vi "Set Cursor Busy.vi"(8 "error in (no error)":errorcluster, 10 "Disable Click?":bool, 11 "IViewable In":refnum<class "IViewable.lvclass">) -> (0 "error out":errorcluster, 3 "IViewable Out":refnum<class "IViewable.lvclass">)   [LabVIEW 2015, in "IViewable.lvlib" / "IViewable.lvclass"]
doc: "<License>\nCopyright © 2017 Composed Systems, LLC | All rights reserved\nwww.composed.io\n\nAuthor: Ethan Stern <ethan.stern@composed.io>\n\nThis software is provided \"AS IS\" WITHOUT WARRANTIES, either express or implied, AND IS FOR EDUCATIONAL PURPOSES ONLY.\n</License>"
uses:
  IViewable.lvclass
  IViewable.lvclass/IViewable.ctl
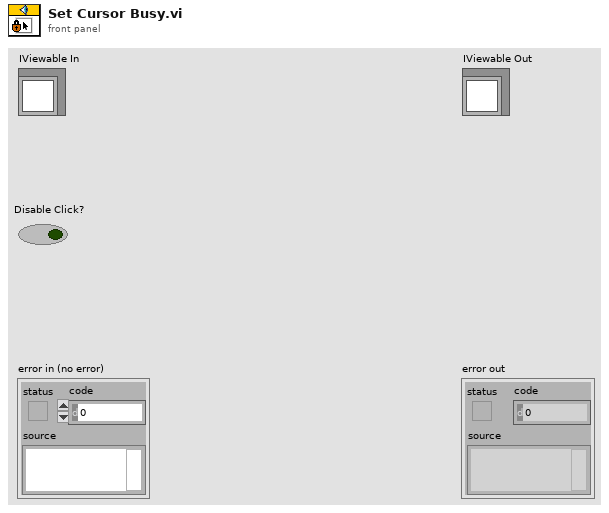
[diagram p1: front panel]
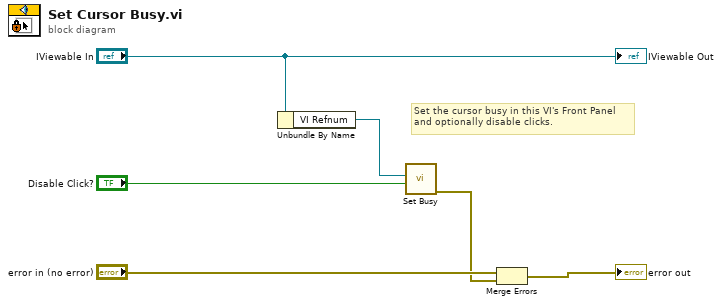
[diagram p0: block diagram]
diagram:
  # "Set the cursor busy in this VI's Front Panel\nand optionally disable clicks."
  n1 = Unbundle By Name("IViewable In") -> ("VI Refnum"=w2:refnum<vi>)
  n2 = call <vilib>:"Set Busy.vi"("disable click? (T)"="Disable Click?", "VI reference (current VI)"=w2) -> ("error out"=w1:errorcluster)  [unwired: 8 in, 1 out]
  n3 = Merge Errors("error in (no error)", w1) -> (→"error out":errorcluster)
  "IViewable Out" <- "IViewable In"
